vi "compLatInc.vi"(1 "FOV":dbl, 2 "% overlap":i32) -> (0 "lat inc. (mm)":dbl)   [LabVIEW 2015]
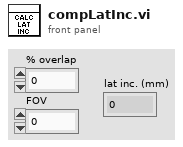
[diagram p1: front panel]
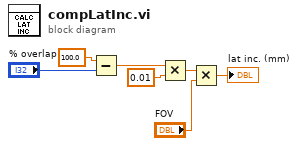
[diagram p0: block diagram]
diagram:
  n1 = Subtract(x=100.0, y="% overlap") -> (x-y=w5:dbl)
  n2 = Multiply(x=w5, y=0.01) -> (x*y=w3:dbl)
  n3 = Multiply(x=w3, y="FOV") -> (x*y=→"lat inc. (mm)":dbl)
